vi "act-0003-cor.vi"   [LabVIEW 2010]
panel:
  # "il n'y a pas d'objets en face-avant : exécutez juste le VI"
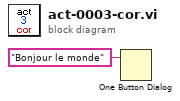
[diagram p0: block diagram]
diagram:
  n1 = One Button Dialog(message="Bonjour le monde") -> ()  [unwired: 1 in, 1 out]
